vi "SetBasePrices.vi"(8 "error in":errorcluster, 11 "Cycles":T1 {"HIGH" min=0.0 max=9.75 step=0.25; "MEDIUM" min=0.0 max=9.75 step=0.25; "LOW" min=0.0 max=9.75 step=0.25; "DELICATE" min=0.0 max=9.75 step=0.25}) -> (0 "error out":errorcluster, 3 "PriceData":string)   [LabVIEW 2023]
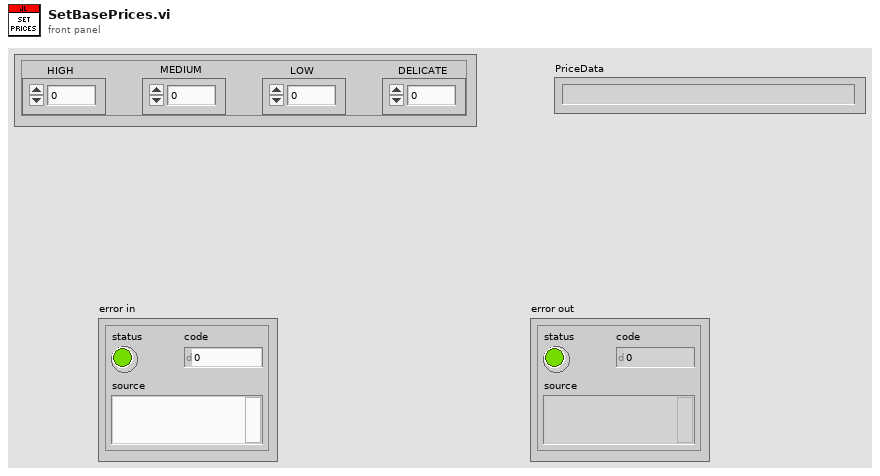
[diagram p1: front panel]
types:
  T1 = cluster{"DELICATE":dbl, "LOW":dbl, "MEDIUM":dbl, "HIGH":dbl}
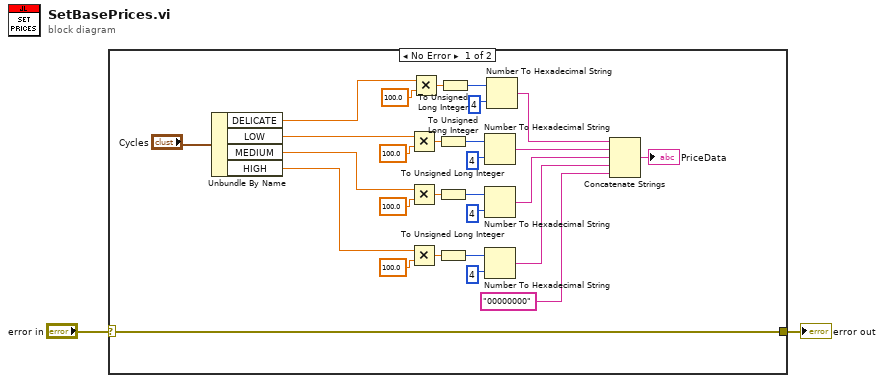
[diagram p0: block diagram]
diagram:
  n1 = case shown="No Error" "error in" {
    selector: "error in" -> [w3 w31]
    tunnel: [w3 w31] -> w1
    frame No Error {
      n2 = Unbundle By Name("Cycles") -> ("DELICATE"=w7:dbl, "LOW"=w6:dbl, "MEDIUM"=w5:dbl, "HIGH"=w4:dbl)
      n3 = Multiply(x=w6, y=100.0) -> (x*y=w25:dbl)
      n4 = Multiply(x=w5, y=100.0) -> (x*y=w20:dbl)
      n5 = Multiply(x=w4, y=100.0) -> (x*y=w17:dbl)
      n6 = Multiply(x=w7, y=100.0) -> (x*y=w28:dbl)
      n7 = To Unsigned Long Integer(number=w25) -> (unsigned 32bit integer=w26:u32)
      n8 = To Unsigned Long Integer(number=w20) -> (unsigned 32bit integer=w19:u32)
      n9 = To Unsigned Long Integer(number=w17) -> (unsigned 32bit integer=w18:u32)
      n10 = To Unsigned Long Integer(number=w28) -> (unsigned 32bit integer=w27:u32)
      n11 = Number To Hexadecimal String(1:i16 4 ("width (-)"), 2:w26) -> (0:w13:string)
      n12 = Number To Hexadecimal String(1:i16 4 ("width (-)"), 2:w19) -> (0:w12:string)
      n13 = Number To Hexadecimal String(1:i16 4 ("width (-)"), 2:w18) -> (0:w11:string)
      n14 = Number To Hexadecimal String(1:i16 4 ("width (-)"), 2:w27) -> (0:w14:string)
      n15 = Concatenate Strings(w14, w13, w12, w11, "00000000" ("string")) -> (→"PriceData":string)
    }
    frame Error {
    }
  }
  "error out" <- w1
